vi "Calcula_CRC.vi"(4 "Message Data":u8[](array[numeric]) format="%.0x") -> (0 "Calculated CRC":u16 format="%.0x", 1 "String":string)   [LabVIEW 2017]
panel:
  out "Send message":u8[](array[numeric]) format="%.0x"
  out "CRC HB":u16 format="%.0x"
  out "CRC LB":u16 format="%.0x"
  in  "Increment":u16=1
  out "Message Length":u16
  # "Bytes + 2"
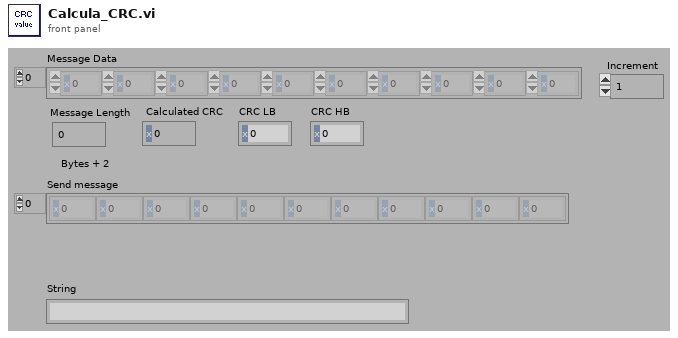
[diagram p1: front panel]
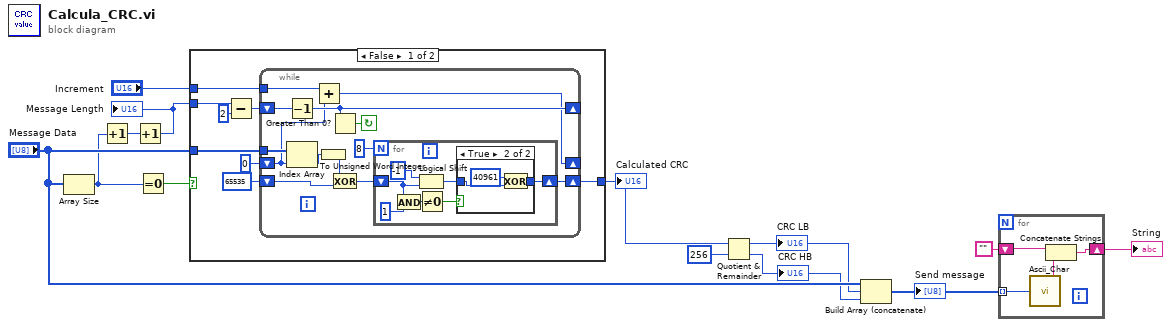
[diagram p0: block diagram]
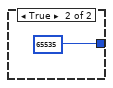
[diagram p3: hidden frame]
diagram:
  n1 = Array Size(array="Message Data") -> (size(s)=w4:i32)
  n2 = Increment(x=w4) -> (x+1=w6:i32)
  n3 = Increment(x=w6) -> (x+1=w5:i32)
  "Message Length" <- w5
  n4 = Equal To 0?(x=w4) -> (x = 0?=w12:bool)
  n5 = case shown="False" w12 {
    tunnel: "Message Data" -> [w21 _]
    tunnel: [w20 u16 65535] -> w11
    tunnel: "Increment" -> [w19 _]
    tunnel: w5 -> [w15 _]
    frame False {
      n6 = Subtract(x=w15, y=u16 2) -> (x-y=w14:i32)
      n7 = while {
        tunnel: w19 -> [w28]
        shift-left: u16 65535 -> [w30]
        shift-right: [w22] -> w20
        tunnel: w21 -> [w31]
        shift-left: u16 0 -> [w27]
        shift-right: [w26] -> _
        shift-left: w14 -> [w34]
        shift-right: [w33] -> _
        stop <- w32 continue-if-true
        n8 = Decrement(x=w34) -> (x-1=w33:i32)
        n9 = Index Array(array=w31, index=w27) -> (element=w25:u8)
        n10 = Add(x=w28, y=w27) -> (x+y=w26:u16)
        n11 = To Unsigned Word Integer(number=w25) -> (unsigned 16bit integer=w24:u16)
        n12 = Greater Than 0?(x=w33) -> (x > 0?=w32:bool)
        n13 = Exclusive Or(1:w30, 2:w24) -> (0:w23:u16)
        n14 = for {
          N: 8 -> [_]
          shift-right: [w35] -> w22
          shift-left: w23 -> [w36]
          n15 = And(x=w36, y=u16 1) -> (x .and. y?=w38:u16)
          n16 = Logical Shift(y=-1, x=w36) -> (x << y=w37:u16)
          n17 = Not Equal To 0?(x=w38) -> (x != 0?=w39:bool)
          n18 = case shown="True" w39 {
            tunnel: [w42 w43] -> w35
            tunnel: w37 -> [w42 w44]
            frame False {
            }
            frame True {
              n19 = Exclusive Or(1:w44, 2:u16 40961) -> (0:w43:u16)
            }
          }
        }
      }
    }
    frame True {
    }
  }
  "Calculated CRC" <- w11
  n20 = Quotient & Remainder(x=w11, y=u16 256) -> (x-y*floor(x/y)=w3:u16, floor(x/y)=w8:u16)
  "CRC LB" <- w3
  "CRC HB" <- w8
  n21 = Build Array (concatenate)("Message Data", w3, w8) -> (w7:u16[])
  "Send message" <- w7
  n22 = for {
    tunnel: w7 -> [w50] mode=indexing
    shift-right: [w48] -> w1
    shift-left: "" -> [w47]
    n23 = call "Ascii_Char.vi"("number"=w50) -> ("ascii char"=w49:string)
    n24 = Concatenate Strings(w47, w49) -> (w48:string)
  }
  "String" <- w1
